vi "Remove Remote Terminal.vi"(8 "error in":errorcluster, 11 "remote terminal":T1 format="%.0x") -> (0 "error out":errorcluster)   [LabVIEW 2020, in "AIM MIL-STD-1553 Scripting.lvlib"]
doc: "Removes the specified <b>remote terminal</b> from the Ballard MIL-STD-1553 system definition. Once the remote terminal has been removed, the <b>remote terminal</b> reference is no longer valid. This VI will return an error if called to remove an invalid <b>remote terminal</b> reference."
uses:
  AIM MIL-STD-1553 Scripting.lvlib
  <vilib>/NI VeriStand/Custom Device API/Custom Device API.lvlib
  <vilib>/NI VeriStand/Custom Device API/Custom Device Item Ref.ctl
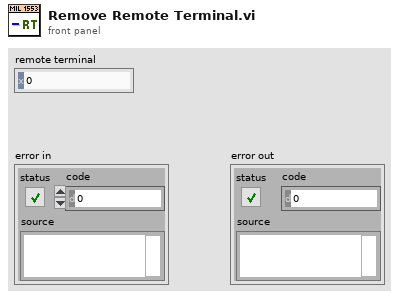
[diagram p1: front panel]
types:
  T1 = typedef "Custom Device API.lvlib/Custom Device Item Ref.ctl" = u64
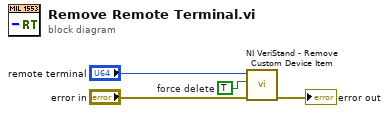
[diagram p0: block diagram]
diagram:
  w4 = TRUE  # force delete
  n1 = call <vilib>:"NI VeriStand - Remove Custom Device Item.vi"("error in (no error)"="error in", "Force Delete (F)"=w4, "Item Ref in"="remote terminal") -> ("error out"=→"error out":errorcluster)  [unwired: 7 in, 1 out]
